vi "WriteToSpreadsheetFile.vi"(4 "Format(%s)":string, 5 "Delimiter(\\t)":string, 6 "Append?(NewFile:F)":bool, 7 "Prompt":string, 8 "ErrorIn":errorcluster, 9 "1D-Data":string[](array[string]), 10 "2D-Data":string[][](array[string]), 11 "FilePath(DialogIfEmpty)":path) -> (0 "ErrorOut":errorcluster, 3 "NewFilePath":path)   [LabVIEW 2018]
doc: "Converts a 2D or 1D array of single-precision numbers to a text string and writes the string to a new byte stream file or appends the string to an existing file.\n\nCopyright © 2011 Epimedia, Inc. All Rights Reserved.\n\nThe Epimedia Application Library is Copyright © 2009-2011 Epimedia, Inc. \nAll Rights Reserved. Used under license."
panel:
  # "Copyright © 2011 Epimedia, Inc. All Rights Reserved.\n\nThe Epimedia Application Library is Copyright © 2009-2011 Epimedia, Inc. \nAll Rights Reserved. Used under license."
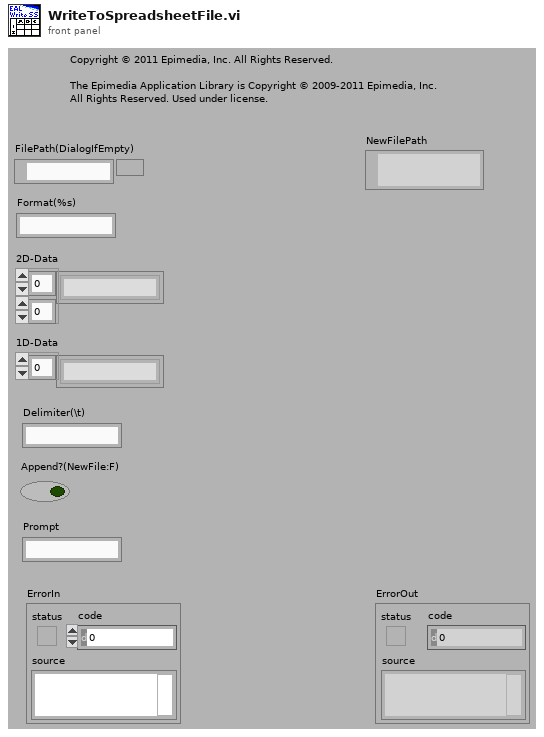
[diagram p1: front panel]
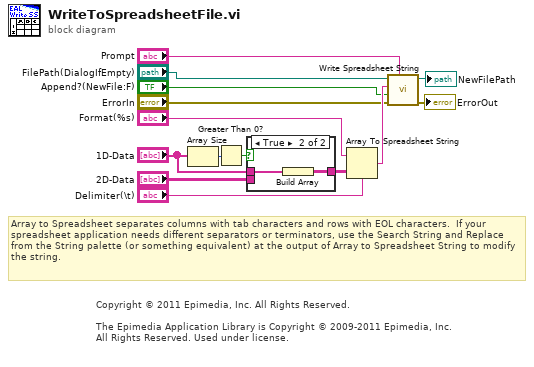
[diagram p0: block diagram]
diagram:
  # "Copyright © 2011 Epimedia, Inc. All Rights Reserved.\n\nThe Epimedia Application Library is Copyright © 2009-2011 Epimedia, Inc. \nAll Rights Reserved. Used under license."
  # "Array to Spreadsheet separates columns with tab characters and rows with EOL characters.  If your spreadsheet application needs different separators or terminators, use the Search String and Replace from the String palette (or something equivalent) at the output of Array to Spreadsheet String to modify the string."
  n1 = Array Size(array="1D-Data") -> (size(s)=w11:i32)
  n2 = Greater Than 0?(x=w11) -> (x > 0?=w12:bool)
  n3 = case shown="True" w12 {
    tunnel: "1D-Data" -> [_ w17]
    tunnel: [w15 w16] -> w13
    tunnel: "2D-Data" -> [w15 _]
    frame False {
    }
    frame True {
      n4 = Build Array(w17) -> (w16:string[][])
    }
  }
  n5 = Array To Spreadsheet String(delimiter (Tab)="Delimiter(\\t)", array=w13, 3:"Format(%s)") -> (spreadsheet string=w14:string)
  n6 = call <vilib>:"Write Spreadsheet String.vi"("prompt"="Prompt", "error in"="ErrorIn", "append to file? (new file:F)"="Append?(NewFile:F)", "spreadsheet string"=w14, "file path (dialog if empty)"="FilePath(DialogIfEmpty)") -> ("error out"=→"ErrorOut":errorcluster, "path"=→"NewFilePath":path)  [unwired: 5 out]
